vi "MListbox Clear Column.vi"(8 "error in (no error)":errorcluster, 10 "Column Inex":u16=4, 11 "Multicolumn ListBox in":refnum<class "Multicolumn ListBox.lvclass">) -> (0 "error out":errorcluster, 3 "Multicolumn ListBox out":refnum<class "Multicolumn ListBox.lvclass">)   [LabVIEW 2012, in "Multicolumn ListBox.lvclass"]
uses:
  Multicolumn ListBox.lvclass
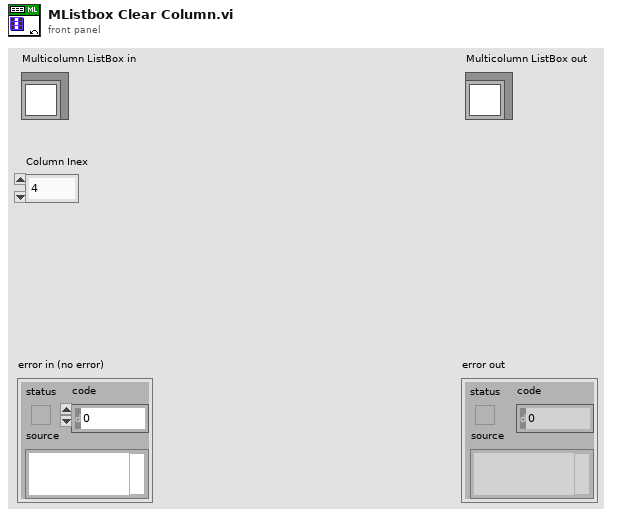
[diagram p1: front panel]
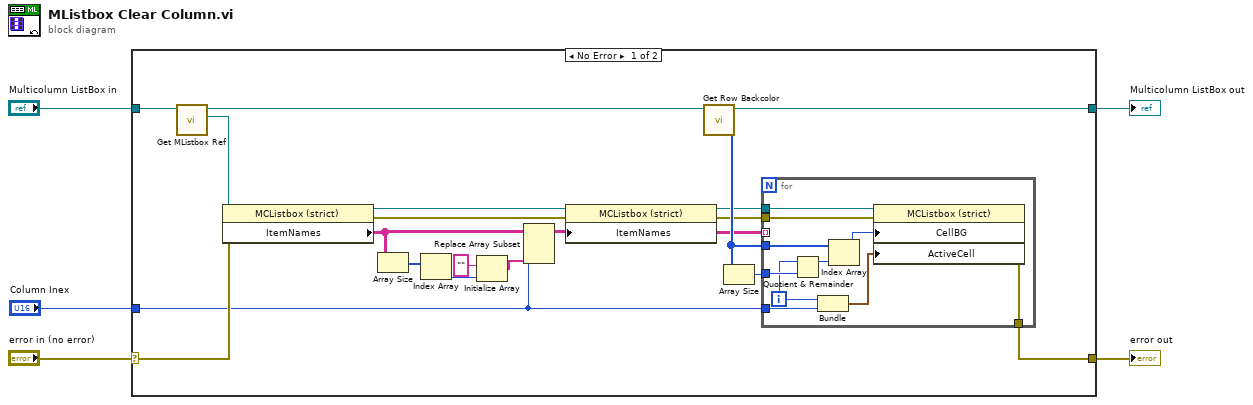
[diagram p0: block diagram]
diagram:
  n1 = case shown="No Error" "error in (no error)" {
    selector: "error in (no error)" -> [w22 w36]
    tunnel: [w18 w36] -> w4
    tunnel: [w19 w35] -> w2
    tunnel: "Multicolumn ListBox in" -> [w24 w35]
    tunnel: "Column Inex" -> [w17 _]
    frame No Error {
      n2 = call "Get MListbox Ref.vi"("Multicolumn ListBox in"=w24) -> ("MListbox Ref"=w23:refnum<vi>, "Multicolumn ListBox out"=w20:refnum<class "Multicolumn ListBox.lvclass">)  [unwired: 8 in, 1 out]
      n3 = property class="MCListbox (strict)"(reference=w23, error in=w22) -> (reference out=w14:refnum<vi>, error out=w16:errorcluster, "ItemNames"=w10:string[][])
      n4 = Array Size(array=w10) -> (size(s)=w9:i32[])
      n5 = Index Array(array=w9) -> (element=w8:i32)  [unwired: 1 in]
      n6 = Initialize Array("", w8) -> (w6:string[])
      n7 = Replace Array Subset(array=w10, new element=w6, index (col)=w17) -> (w12:string[][])  [unwired: 1 in]
      n8 = property class="MCListbox (strict)"(reference=w14, error in=w16, "ItemNames"=w12) -> (reference out=w13:refnum<vi>, error out=w15:errorcluster)
      n9 = call "Get Row Backcolor.vi"("Multicolumn ListBox in"=w20) -> ("Row Backcolor"=w21:u32[], "Multicolumn ListBox out"=w19:refnum<class "Multicolumn ListBox.lvclass">)  [unwired: 8 in, 1 out]
      n10 = Array Size(array=w21) -> (size(s)=w11:i32)
      n11 = for {
        tunnel: w12 -> [_] mode=indexing
        tunnel: w13 -> [w31]
        tunnel: w11 -> [w34]
        tunnel: w21 -> [w33]
        tunnel: w15 -> [w27]
        tunnel: [w26] -> w18
        tunnel: w17 -> [w25]
        i -> [w29]
        n12 = Quotient & Remainder(x=w29, y=w34) -> (x-y*floor(x/y)=w32:i32)  [unwired: 1 out]
        n13 = Bundle(w29, "Column Inex"=w25) -> (w28:cluster{i32, "Column Inex":u16})  [unwired: 1 in]
        n14 = Index Array(array=w33, index=w32) -> (element=w30:u32)
        n15 = property class="MCListbox (strict)"(reference=w31, error in=w27, "CellBG"=w30, "ActiveCell"=w28) -> (error out=w26:errorcluster)  [unwired: 1 out]
      }
    }
    frame Error {
    }
  }
  "error out" <- w4
  "Multicolumn ListBox out" <- w2
